vi "BuildCommand.vi"(4 "ReadLength (bytes) in":u8, 5 "ReplyType [7-bit]":T4=enum."7-bit", 6 "Register":u8 format="%.0x", 7 "AddressType [14-bit]":T1, 9 "Argument":i32 format="%02x", 10 "CommandDescriptor":T2={"PololuCommand"="ReadModeStatus", "Mnemonic"="", "CommandType"=enum."Command", "Min"=0, "Max"=0}, 11 "Address":u16=16384 caption="Address [16384= Unadressed]") -> (1 "ReadLength (bytes) out":u8, 2 "AssembledCommand":string)   [LabVIEW 2021]
uses:
  TicReplyStyle.ctl
  PololuCommandDescriptor.ctl
  TicCommandType.ctl
  TicAddressStyle.ctl
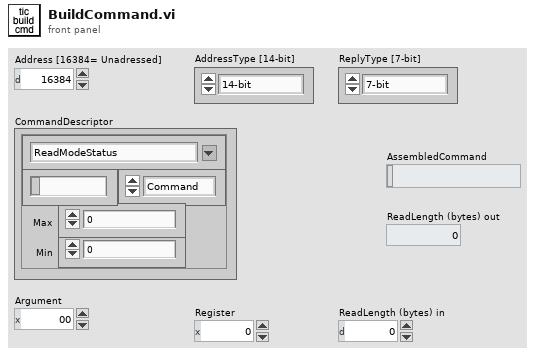
[diagram p1: front panel]
types:
  T1 = typedef "TicAddressStyle.ctl" = enum16{"14-bit", "7-bit"}
  T2 = typedef "PololuCommandDescriptor.ctl" = cluster{"PololuCommand":string, "Mnemonic":string, "CommandType":T3, "Min":i32, "Max":i32}
  T3 = typedef "TicCommandType.ctl" = enum16{"Command", "7-bitWrite", "32-bitWrite", "BlockRead"}
  T4 = typedef "TicReplyStyle.ctl" = enum16{"8-bit", "7-bit"}
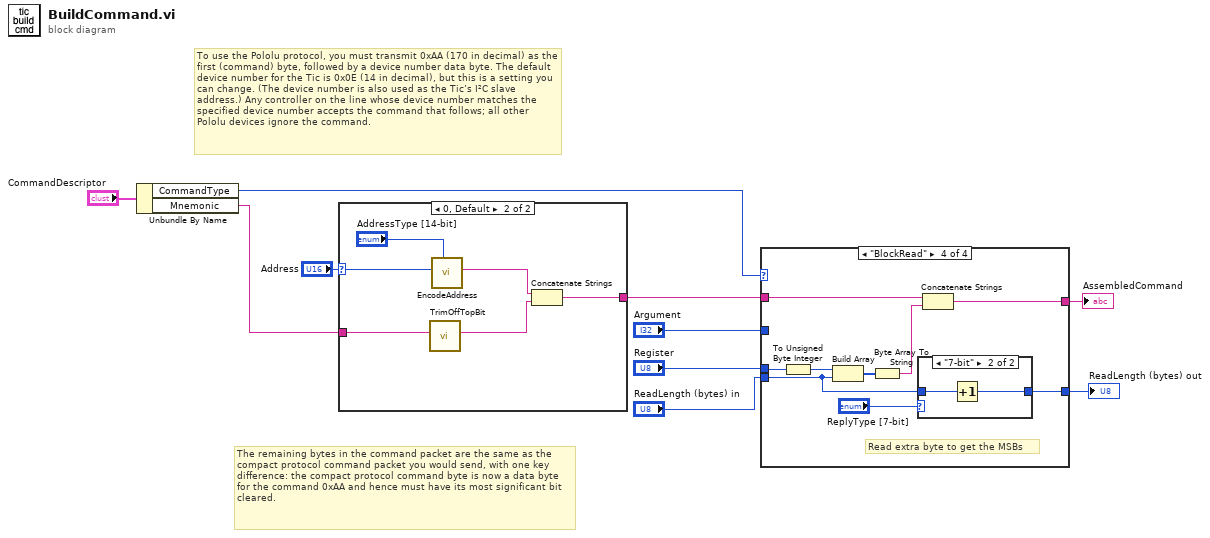
[diagram p0: block diagram]
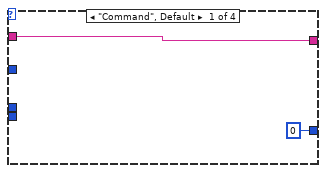
[diagram p3: hidden frame]
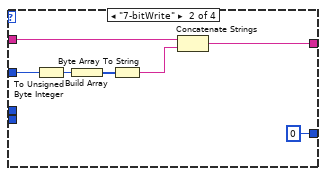
[diagram p4: hidden frame]
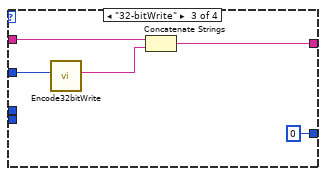
[diagram p5: hidden frame]
diagram:
  # "The remaining bytes in the command packet are the same as the compact protocol command packet you would send, with one key difference: the compact protocol command byte is now a data byte for the command 0xAA and hence must have its most significant bit cleared."
  # "To use the Pololu protocol, you must transmit 0xAA (170 in decimal) as the first (command) byte, followed by a device number data byte. The default device number for the Tic is 0x0E (14 in decimal), but this is a setting you can change. (The device number is also used as the Tic’s I²C slave address.) Any controller on the line whose device number matches the specified device number accepts the command that follows; all other Pololu devices ignore the command."
  n1 = Unbundle By Name("CommandDescriptor") -> ("CommandType"=w2:T3, "Mnemonic"=w1:string)
  n2 = case shown="0, Default" "Address" {
    selector: "Address" -> [_ w17]
    tunnel: [w11 w15] -> w4
    tunnel: w1 -> [w11 w13]
    frame 16384 {
    }
    frame 0, Default {
      n3 = call "TrimOffTopBit.vi"("8bitMnemonic in"=w13) -> ("7bitMnemonic"=w14:string)  [unwired: 10 in]
      n4 = call "EncodeAddress.vi"("AddressType"="AddressType [14-bit]", "Address"=w17) -> ("PololuAddressString"=w16:string)  [unwired: 9 in]
      n5 = Concatenate Strings(w16, w14) -> (w15:string)
    }
  }
  n6 = case shown="\"BlockRead\"" w2 {
    tunnel: "Register" -> [_ _ _ w40]
    tunnel: w4 -> [w19 w24 w31 w37]
    tunnel: [w19 w22 w29 w35] -> w5
    tunnel: "ReadLength (bytes) in" -> [_ _ _ w33]
    tunnel: "Argument" -> [_ w21 w28 _]
    tunnel: [u8 0 ("ReadLength (bytes)") u8 0 ("ReadLength (bytes)") u8 0 ("ReadLength (bytes)") w32] -> w10
    frame "Command", Default {
    }
    frame "7-bitWrite" {
      n7 = To Unsigned Byte Integer(number=w21) -> (unsigned 8bit integer=w26:u8)
      n8 = Build Array(w26) -> (w25:u8[])
      n9 = Byte Array To String(unsigned byte array=w25) -> (string=w23:string)
      n10 = Concatenate Strings(w24, w23) -> (w22:string)
    }
    frame "32-bitWrite" {
      n11 = call "Encode32bitWrite.vi"("Numeric"=w28) -> ("PololuString"=w30:string)  [unwired: 10 in]
      n12 = Concatenate Strings(w31, w30) -> (w29:string)
    }
    frame "BlockRead" {
      # "Read extra byte to get the MSBs"
      n13 = To Unsigned Byte Integer(number=w40) -> (unsigned 8bit integer=w39:u8)
      n14 = Build Array(w39, w33) -> (w38:u8[])
      n15 = Byte Array To String(unsigned byte array=w38) -> (string=w36:string)
      n16 = case shown="\"7-bit\"" "ReplyType [7-bit]" {
        tunnel: w33 -> [w41 w43]
        tunnel: [w41 w42] -> w32
        frame "8-bit", Default {
        }
        frame "7-bit" {
          n17 = Increment(x=w43) -> (x+1=w42:u8)
        }
      }
      n18 = Concatenate Strings(w37, w36) -> (w35:string)
    }
  }
  "ReadLength (bytes) out" <- w10
  "AssembledCommand" <- w5
